vi "Drive Loop Cheesey Drive.vi"(9 "Wheel":dbl, 10 "Throttle":dbl, 11 "Drive Loop Cluster":T1) -> ()   [LabVIEW 2015]
uses:
  Drive Code Bundle.ctl
  Sensor Cluster.ctl
  Camera Cluster.ctl
  Drive Code Notifier.ctl
  Drive Code Command.ctl
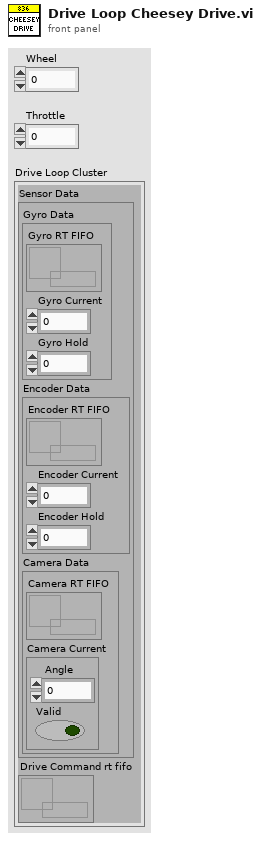
[diagram p1: front panel]
types:
  T1 = typedef "Drive Code Bundle.ctl" = cluster{"Sensor Data":T2, "Drive Command rt fifo":refnum<k33>}
  T2 = typedef "Sensor Cluster.ctl" = cluster{"Gyro Data":cluster{"Gyro RT FIFO":refnum<k33>, "Gyro Current":dbl, "Gyro Hold":dbl}, "Encoder Data":cluster{"Encoder RT FIFO":refnum<k33>, "Encoder Current":dbl, "Encoder Hold":dbl}, "Camera Data":cluster{"Camera RT FIFO":refnum<k33>, "Camera Current":T3}}
  T3 = typedef "Camera Cluster.ctl" = cluster{" Angle":dbl, "Valid":bool}
  T4 = typedef "Drive Code Command.ctl" = enum16{"Do Nothing", "Manual", "Drive Continuous", "Turn", "Drive Distance", "Hold Position", "Hold Yaw", "Follow Camera", "Turn to Camera"}
  T5 = typedef "Drive Code Notifier.ctl" = cluster{"Command":T4, "Parameter A":dbl, "Parameter B":dbl, "Parameter C":dbl, "Absolute?":bool}
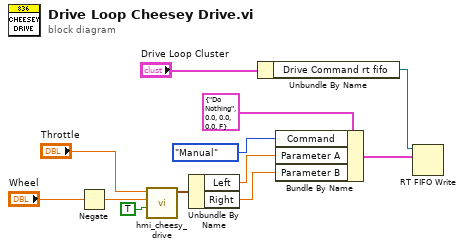
[diagram p0: block diagram]
diagram:
  n1 = Negate(x="Wheel") -> (-x=w6:dbl)
  n2 = call <userlib>:"hmi_cheesy_drive.vi"("Quick Turn"=TRUE, "Wheel"=w6, "Throttle"="Throttle") -> ("Drive Data"=w7:cluster{"Left":dbl, "Right":dbl})  [unwired: 8 in]
  n3 = Unbundle By Name(w7) -> ("Left"=w8:dbl, "Right"=w9:dbl)
  n4 = Unbundle By Name("Drive Loop Cluster") -> ("Drive Command rt fifo"=w12:refnum<k33>)
  n5 = Bundle By Name(cluster=T5 {"Command"=enum."Do Nothing", "Parameter A"=0.0, "Parameter B"=0.0, "Parameter C"=0.0, "Absolute?"=FALSE}, "Command"=Drive_Code_Command."Manual", "Parameter A"=w8, "Parameter B"=w9) -> (w11:T5)
  n6 = RT FIFO Write(0:w12, 1:w11) -> ()  [unwired: 3 in, 4 out]
